vi "sliderMove.vi"(1 "position":u16(ring) items=["0", "1", "2", "3"]) -> (0 "success":bool)   [LabVIEW 2017]
uses:
  <vilib>/Instr/_visa.llb/VISA Flush IO Buffer Mask.ctl
  globalDevices.vi
panel:
  out "read buffer":string
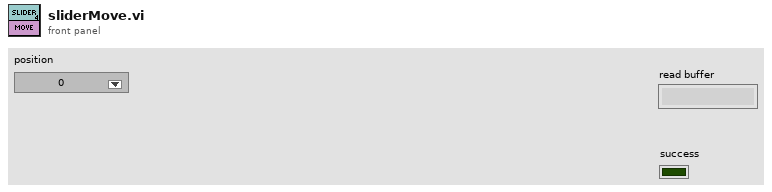
[diagram p1: front panel]
types:
  T1 = typedef "VISA Flush IO Buffer Mask.ctl" = u16
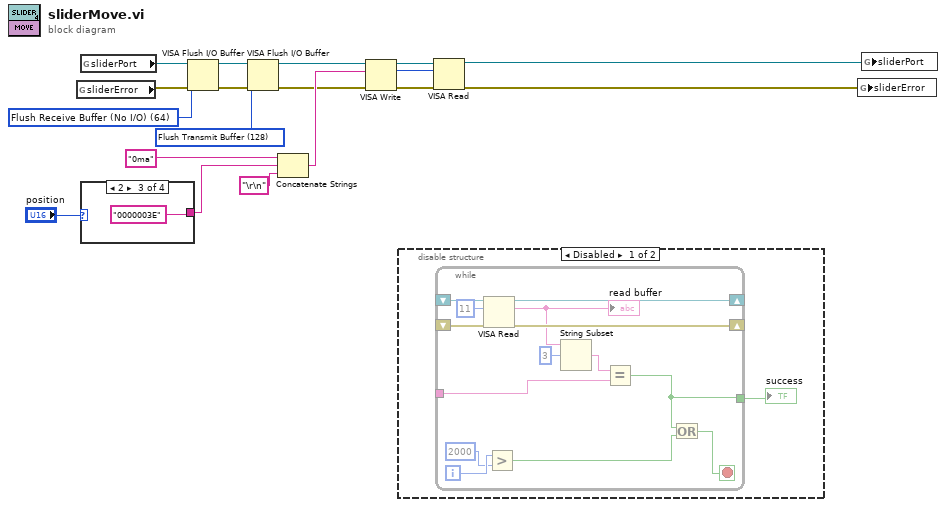
[diagram p0: block diagram]
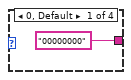
[diagram p3: hidden frame]
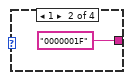
[diagram p4: hidden frame]
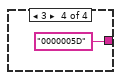
[diagram p5: hidden frame]
diagram:
  w1 = T1 128 items=["Flush Receive Buffer"=16, "Write Transmit Buffer to Device"=32, "Flush Receive Buffer (No I/O)"=64, "Flush Transmit Buffer"=128] ("Mask")
  w6 = T1 64 items=["Flush Receive Buffer"=16, "Write Transmit Buffer to Device"=32, "Flush Receive Buffer (No I/O)"=64, "Flush Transmit Buffer"=128] ("Mask")
  n1 = global read "globalDevices.vi" "sliderError"() -> (w12:errorcluster)
  n2 = global read "globalDevices.vi" "sliderPort"() -> (w13:refnum<visa-resource-name>)
  n3 = case shown="2" "position" {
    tunnel: ["00000000" "0000001F" "0000003E" "0000005D"] -> w14
    frame 0, Default {
    }
    frame 1 {
    }
    frame 2 {
    }
    frame 3 {
    }
  }
  n4 = VISA Flush I/O Buffer(VISA resource name=w13, mask (16)=w6, error in (no error)=w12) -> (VISA resource name out=w4:refnum<visa-resource-name>, error out=w5:errorcluster)
  n5 = VISA Flush I/O Buffer(VISA resource name=w4, mask (16)=w1, error in (no error)=w5) -> (VISA resource name out=w3:refnum<visa-resource-name>, error out=w2:errorcluster)
  n6 = Concatenate Strings("0ma", w14, "\r\n" ("string")) -> (w16:string)
  n7 = VISA Write(VISA resource name=w3, write buffer=w16, error in (no error)=w2) -> (VISA resource name out=w11:refnum<visa-resource-name>, return count=w10:u32, error out=w9:errorcluster)
  n8 = disable-structure shown="Disabled" {
    frame Disabled {
      n9 = while {
        shift-right: [w35] -> _
        shift-left: _ -> [w37]
        shift-right: [w34] -> _
        shift-left: _ -> [w36]
        tunnel: _ -> [w29]
        tunnel: [w24] -> w23
        i -> [w28]
        stop <- w25 stop-if-true
        n10 = VISA Read(VISA resource name=w37, byte count=u32 11, error in (no error)=w36) -> (VISA resource name out=w35:refnum<visa-resource-name>, read buffer=w32:string, error out=w34:errorcluster)  [unwired: 1 out]
        "read buffer" <- w32
        n11 = Greater?(x=w28, y=2000) -> (0:w26:bool)
        n12 = String Subset(string=w32, offset (0)=3) -> (substring=w30:string)  [unwired: 1 in]
        n13 = Equal?(x=w30, y=w29) -> (x = y?=w24:bool)
        n14 = Or(x=w24, y=w26) -> (x .or. y?=w25:bool)
      }
      "success" <- w23
    }
    frame Enabled {
    }
  }
  n15 = VISA Read(VISA resource name=w11, byte count=w10, error in (no error)=w9) -> (VISA resource name out=w8:refnum<visa-resource-name>, error out=w7:errorcluster)  [unwired: 2 out]
  n16 = global write "globalDevices.vi" "sliderError"(w7) -> ()
  n17 = global write "globalDevices.vi" "sliderPort"(w8) -> ()
